vi "Write Data_Test Database.vi"(8 "error in (no error)":errorcluster caption="entrée d'erreur (pas d'erreur)", 11 "Actor Test Database en entrée":refnum<class "Actor Test Database.lvclass">) -> (0 "error out":errorcluster caption="sortie d'erreur", 3 "Actor Test Database en sortie":refnum<class "Actor Test Database.lvclass">)   [LabVIEW 2020, in "Library Core.lvlib" / "Actor Test Database.lvclass"]
uses:
  Actor Test Database.lvclass
  C:/Users/ngarcin/OneDrive - Altyor/Standard TB/Class/Sequencer/Actor Test (Default)/Actor Test (Default).lvclass
  Database/Database Altyor/Database Altyor.lvclass
  JSON API/JSON Value/Set from JSON string.vi
  JSON API/Variant JSON/Variant to JSON.vi
  JSON API/JSON Value/Get Item by name array.vi
  Sequencer (Default)/Sequencer (Default).lvclass
  Instrument/Instrument (Default)/Class Instrument (Default).lvclass
  JSON API/JSON Value/JSON Value.lvclass
  Actor Test Database.lvclass/Actor Test Database.ctl
  JSON API/Variant JSON/Variant JSON.lvlib
  JSON API/Get Polymorphic/JSON GetSet.lvlib
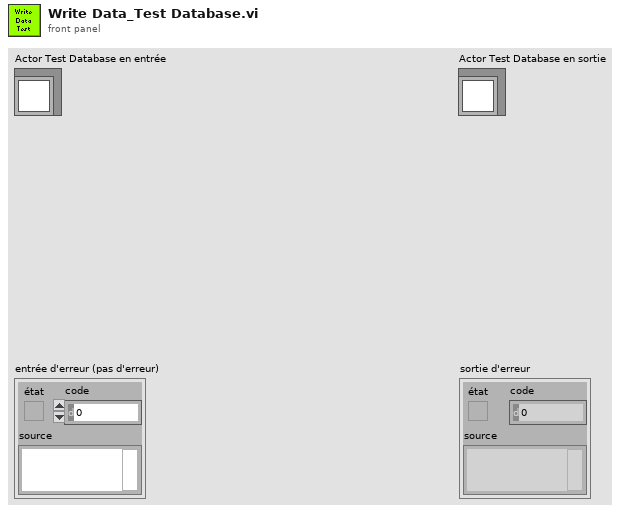
[diagram p1: front panel]
types:
  T1 = cluster{"Connection Name ODBC":string, "DatabaseName":string, "Condition":string, "Type Data ":enum16{"Data Product", "Data Test"}, "Database Altyor":refnum<class "Database Altyor.lvclass">}
  T2 = typedef "Library Commun.lvlib/Commande Value Type.ctl" = enum16{"None", "String", "Number", "Timestamp", "Boolean", "Array"}
  T3 = typedef "Library Commun.lvlib/Commande Type Test.ctl" = enum16{"Function", "Test", "Calculation"}
  T4 = cluster{"Main Test":string, "Name Test":string, "StartOfTest":string, "Value":string, "Limit_Low":string, "Limit_High":string, "Result":bool, "Fatal_Test":bool, "NbRetry":dbl, "EndOfTest":string, "Error":string, "TypeValue":T2, "Type Test":T3}[]
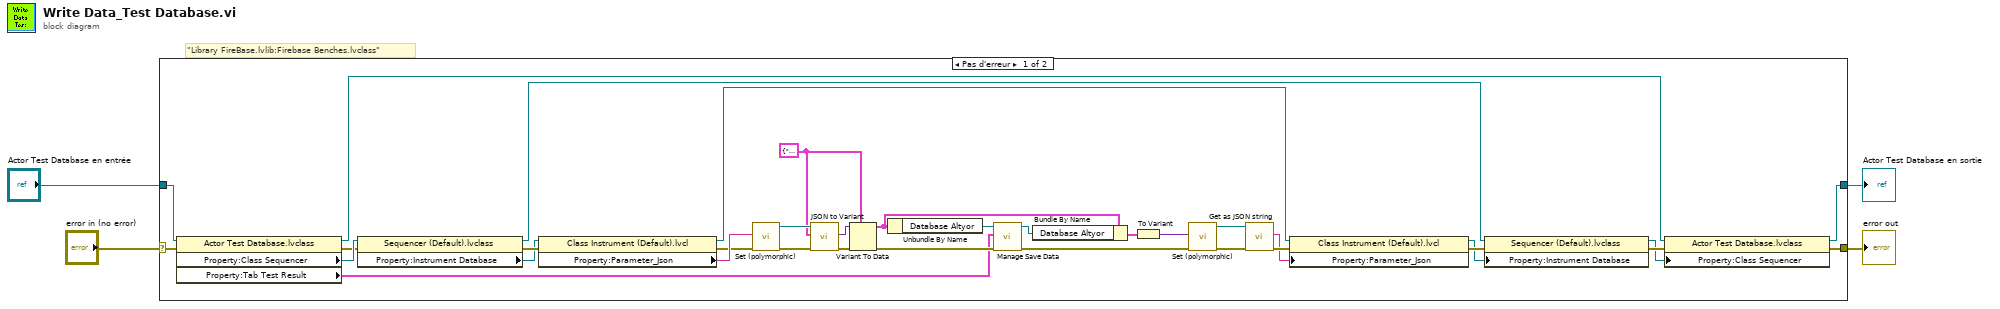
[diagram p0: block diagram]
diagram:
  # "\"Library FireBase.lvlib:Firebase Benches.lvclass\""
  n1 = case shown="Pas d'erreur" "error in (no error)" {
    selector: "error in (no error)" -> [w36 w39]
    tunnel: [w8 w40] -> w2
    tunnel: "Actor Test Database en entrée" -> [w37 w40]
    tunnel: [w10 w39] -> w1
    frame No Error {
      w7 = T1 {"Connection Name ODBC"="", "DatabaseName"="", "Condition"="", "Type Data "=enum."Data Product", "Database Altyor"=refnum} ("Parameter")
      n2 = property class="Actor Test Database.lvclass"(reference=w37, error in=w36) -> (reference out=w11:refnum<class "Actor Test Database.lvclass">, error out=w35:errorcluster, "Property:Class Sequencer"=w38:refnum<class "Sequencer (Default).lvclass">, "Property:Tab Test Result"=w5:T4)
      n3 = property class="Sequencer (Default).lvclass"(reference=w38, error in=w35) -> (reference out=w14:refnum<class "Sequencer (Default).lvclass">, error out=w28:errorcluster, "Property:Instrument Database"=w27:refnum<class "Class Instrument (Default).lvclass">)
      n4 = property class="Class Instrument (Default).lvcl"(reference=w27, error in=w28) -> (reference out=w15:refnum<class "Class Instrument (Default).lvclass">, error out=w29:errorcluster, "Property:Parameter_Json"=w30:string)
      n5 = call-poly "Set (polymorphic).vi"("error in (no error)"=w29, "JSON stream"=w30) -> ("error out"=w32:errorcluster, "JSON Value out"=w34:refnum<class "JSON Value.lvclass">)  [unwired: 7 in, 1 out]
      n6 = call "JSON to Variant.vi"("error in (no error)"=w32, "Variant (Data Type)"=w7, "JSON Value"=w34) -> ("error out"=w33:errorcluster, "Variant out"=w31:variant)  [unwired: 7 in]
      n7 = Variant To Data(error in=w33, type=w7, Variant=w31) -> (data=w9:T1, error out=w6:errorcluster)
      n8 = Unbundle By Name(w9) -> ("Database Altyor"=w26:refnum<class "Database Altyor.lvclass">)
      n9 = call "Manage Save Data.vi"("entrée d'erreur (pas d'erreur)"=w6, "Data"=w5, "Database Altyor En entrée"=w26) -> ("sortie d'erreur"=w16:errorcluster, "Database Altyor En Sortie"=w17:refnum<class "Database Altyor.lvclass">)  [unwired: 7 in]
      n10 = Bundle By Name(cluster=w9, "Database Altyor"=w17) -> (w21:T1)
      n11 = To Variant(anything=w21) -> (Variant=w18:variant)
      n12 = call-poly "Set (polymorphic).vi"("error in (no error)"=w16, "Variant"=w18) -> ("error out"=w20:errorcluster, "JSON Value out"=w19:refnum<class "JSON Value.lvclass">)  [unwired: 8 in]
      n13 = call "Get as JSON string.vi"("error in (no error)"=w20, "JSON Value in"=w19) -> ("error out"=w23:errorcluster, "<JSON>"=w22:string)  [unwired: 8 in]
      n14 = property class="Class Instrument (Default).lvcl"(reference=w15, error in=w23, "Property:Parameter_Json"=w22) -> (reference out=w24:refnum<class "Class Instrument (Default).lvclass">, error out=w25:errorcluster)
      n15 = property class="Sequencer (Default).lvclass"(reference=w14, error in=w25, "Property:Instrument Database"=w24) -> (reference out=w12:refnum<class "Sequencer (Default).lvclass">, error out=w13:errorcluster)
      n16 = property class="Actor Test Database.lvclass"(reference=w11, error in=w13, "Property:Class Sequencer"=w12) -> (reference out=w8:refnum<class "Actor Test Database.lvclass">, error out=w10:errorcluster)
    }
    frame Error {
    }
  }
  "error out" <- w1
  "Actor Test Database en sortie" <- w2
